vi "Disconnect.vi"(8 "error in (no error)":errorcluster, 10 "Params":variant, 11 "PIPXI40 Matrix in":refnum<class "PIPXI40 Matrix.lvclass">) -> (0 "error out":errorcluster, 3 "PIPXI40 Matrix out":refnum<class "PIPXI40 Matrix.lvclass">)   [LabVIEW 2020, in "PIPXI40.lvlib" / "PIPXI40 Matrix.lvclass"]
uses:
  PIPXI40 Matrix.lvclass
  D:/WSGitHub/RTFWK/Realization/PIPXI40 Base/PIPXI40 Base.lvclass
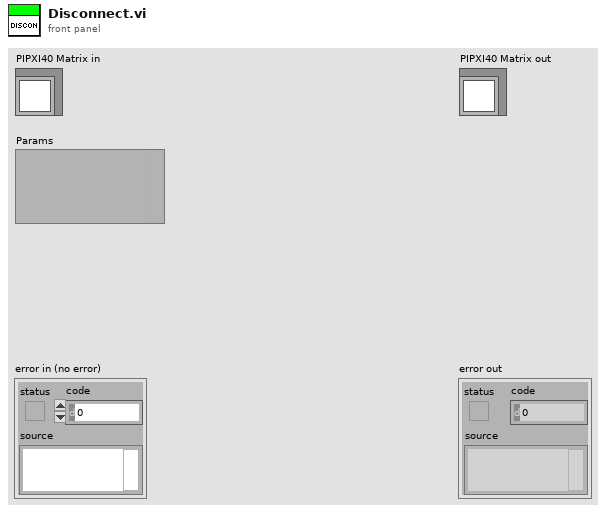
[diagram p1: front panel]
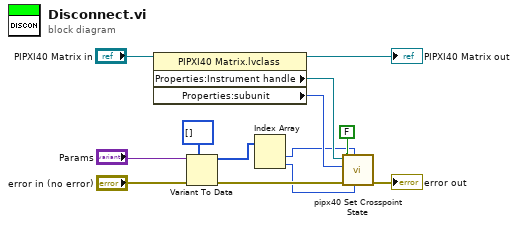
[diagram p0: block diagram]
diagram:
  n1 = property class="PIPXI40 Matrix.lvclass"(reference="PIPXI40 Matrix in") -> (reference out=→"PIPXI40 Matrix out":refnum<class "PIPXI40 Matrix.lvclass">, "Properties:Instrument handle"=w12:refnum<visa-resource-name>, "Properties:subunit"=w13:u32)  [unwired: 1 in, 1 out]
  n2 = Variant To Data(error in="error in (no error)", type=u32[] [], Variant="Params") -> (data=w3:u32[], error out=w10:errorcluster)
  n3 = Index Array(array=w3) -> (element #1=w2:u32, element #2=w1:u32)  [unwired: 2 in]
  n4 = call <instrlib>:"pipx40 Set Crosspoint State.vi"("column location"=w1, "row location"=w2, "error in (no error)"=w10, "action"=FALSE, "subunit number"=w13, "instrument handle"=w12) -> ("error out"=→"error out":errorcluster)  [unwired: 4 in, 1 out]
